vi "receiveInputs.vi"(8 "error in (no error)":errorcluster, 11 "ILC in":refnum<class "ILC.lvclass">) -> (0 "error out":errorcluster, 1 "ADCs in Engineering Units":T1 {"Ch4" format="%.1f"; "Ch3" format="%.1f"; "Ch2" format="%.1f"; "Ch1" format="%.1f"}, 2 "InputData":T2, 3 "ILC out":refnum<class "ILC.lvclass">)   [LabVIEW 2015, in "ILCCommon.lvlib" / "ILC.lvclass"]
uses:
  <userlib>/Common/ILC/ILC/ILC.lvclass
  <userlib>/Common/ILC/Typedefs/ADC Raw.ctl
  <userlib>/Common/ILC/Typedefs/ILCTypedefs.lvlib
  <userlib>/Common/ILC/Typedefs/Limit Switches.ctl
  <userlib>/Common/ILC/Configuration/Input Channels.ctl
  <userlib>/Common/ILC/Configuration/ILCConfiguration.lvlib
  <userlib>/Common/ILC/Typedefs/Inputs.ctl
  <userlib>/Common/ILC/Typedefs/ADC Eng.ctl
panel:
  # "Limit Switches"
  # "ADCs Raw"
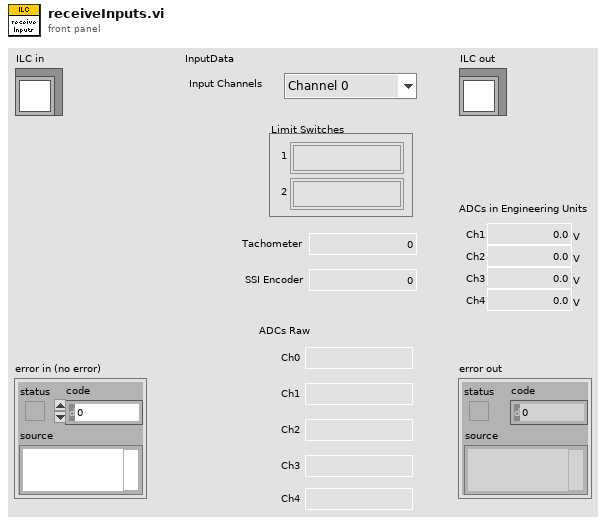
[diagram p1: front panel]
types:
  T1 = typedef "ILCCommon.lvlib/ILCTypedefs.lvlib/ADC Eng.ctl" = cluster{"Ch1":dbl[unit], "Ch2":dbl[unit], "Ch3":dbl[unit], "Ch4":dbl[unit]}
  T2 = typedef "ILCCommon.lvlib/ILCTypedefs.lvlib/Inputs.ctl" = cluster{"Input Channels":T3, "Limit Switches":T4, "Tachometer":u16, "SSI Encoder":i32, "ADC":T5}
  T3 = typedef "ILCCommon.lvlib/ILCConfiguration.lvlib/Input Channels.ctl" = enum16{"Channel 0", "3 Channels", "5 Channels"}
  T4 = typedef "ILCCommon.lvlib/ILCTypedefs.lvlib/Limit Switches.ctl" = cluster{"1":bool, "2":bool}
  T5 = typedef "ILCCommon.lvlib/ILCTypedefs.lvlib/ADC Raw.ctl" = cluster{"Ch0":i32, "Ch1":i32, "Ch2":i32, "Ch3":i32, "Ch4":i32}
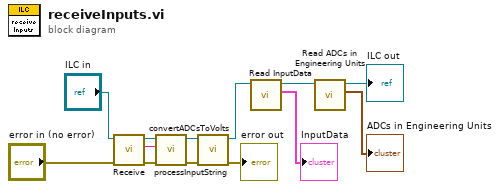
[diagram p0: block diagram]
diagram:
  n1 = call-dynamic "Receive.vi"("error in (no error)"="error in (no error)", "ILC in"="ILC in") -> ("error out"=w4:errorcluster, "Response"=w1:string, "ILC out"=w3:refnum<class "ILC.lvclass">)  [unwired: 7 in]
  n2 = call <userlib>:"processInputString.vi"("error in (no error)"=w4, "stringRead"=w1, "ILC in"=w3) -> ("error out"=w8:errorcluster, "ILC out"=w9:refnum<class "ILC.lvclass">)  [unwired: 7 in]
  n3 = call <userlib>:"convertADCsToVolts.vi"("error in (no error)"=w8, "ILC in"=w9) -> ("error out"=→"error out":errorcluster, "ILC out"=w7:refnum<class "ILC.lvclass">)  [unwired: 8 in]
  n4 = call <userlib>:"Read InputData.vi"("ILC in"=w7) -> ("InputData"=→"InputData":T2, "ILC out"=w13:refnum<class "ILC.lvclass">)  [unwired: 9 in]
  n5 = call <userlib>:"Read ADCs in Engineering Units.vi"("ILC in"=w13) -> ("ADCs in Engineering Units"=→"ADCs in Engineering Units":T1, "ILC out"=→"ILC out":refnum<class "ILC.lvclass">)  [unwired: 9 in]
